vi "Select Element from Array.vi"(0 "Data In":path[](array[path]), 7 "Select?":bool[](array[boolean])) -> (4 "Data Out":path[](array[path]))   [LabVIEW 2010]
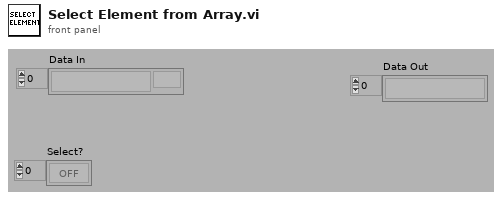
[diagram p1: front panel]
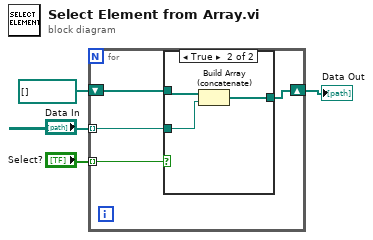
[diagram p0: block diagram]
diagram:
  n1 = for {
    tunnel: "Data In" -> [w6] mode=indexing
    tunnel: "Select?" -> [w8] mode=indexing
    shift-right: [w5] -> w4
    shift-left: path[] [] ("sorted array") -> [w7]
    n2 = case shown="True" w8 {
      tunnel: w7 -> [w9 w12]
      tunnel: w6 -> [_ w11]
      tunnel: [w9 w10] -> w5
      frame False {
      }
      frame True {
        n3 = Build Array (concatenate)(w12, w11) -> (w10:path[])
      }
    }
  }
  "Data Out" <- w4
